vi "TEST.vi"() -> ()   [LabVIEW 2015, in "Copy of Untitled Library 1.lvlib"]
uses:
  Copy of Untitled Library 1.lvlib
  <userlib>/origin_lib_main/userlogin_lib/Control/Queue and Caller MSG.ctl
  Controls/Control 1.ctl
  <vilib>/addons/database/Connection.llb/DB Tools Open Connec (String).vi
  API/Init Module.vi
  API/Get Open batch .vi
  Main.vi
  <vilib>/addons/database/NI_Database_API.lvlib
panel:
  out "subarray":string[](array[string])
  in  "Get Open Batch data":bool
  out "Batch Data 3":T1
  out "Module Number 2":dbl
  out "Product name":string
  out "UI Controllers":string[](array[string])
  out "Enum":T2(ring)
  in  "stop 2":bool
  in  "Init":bool
  in  "Module Number":dbl=1.0
  in  "Main":bool
  in  "stop":bool
  out "error out":errorcluster
  in  "UI COnfiguration  2":T4
  # "QUEUE"
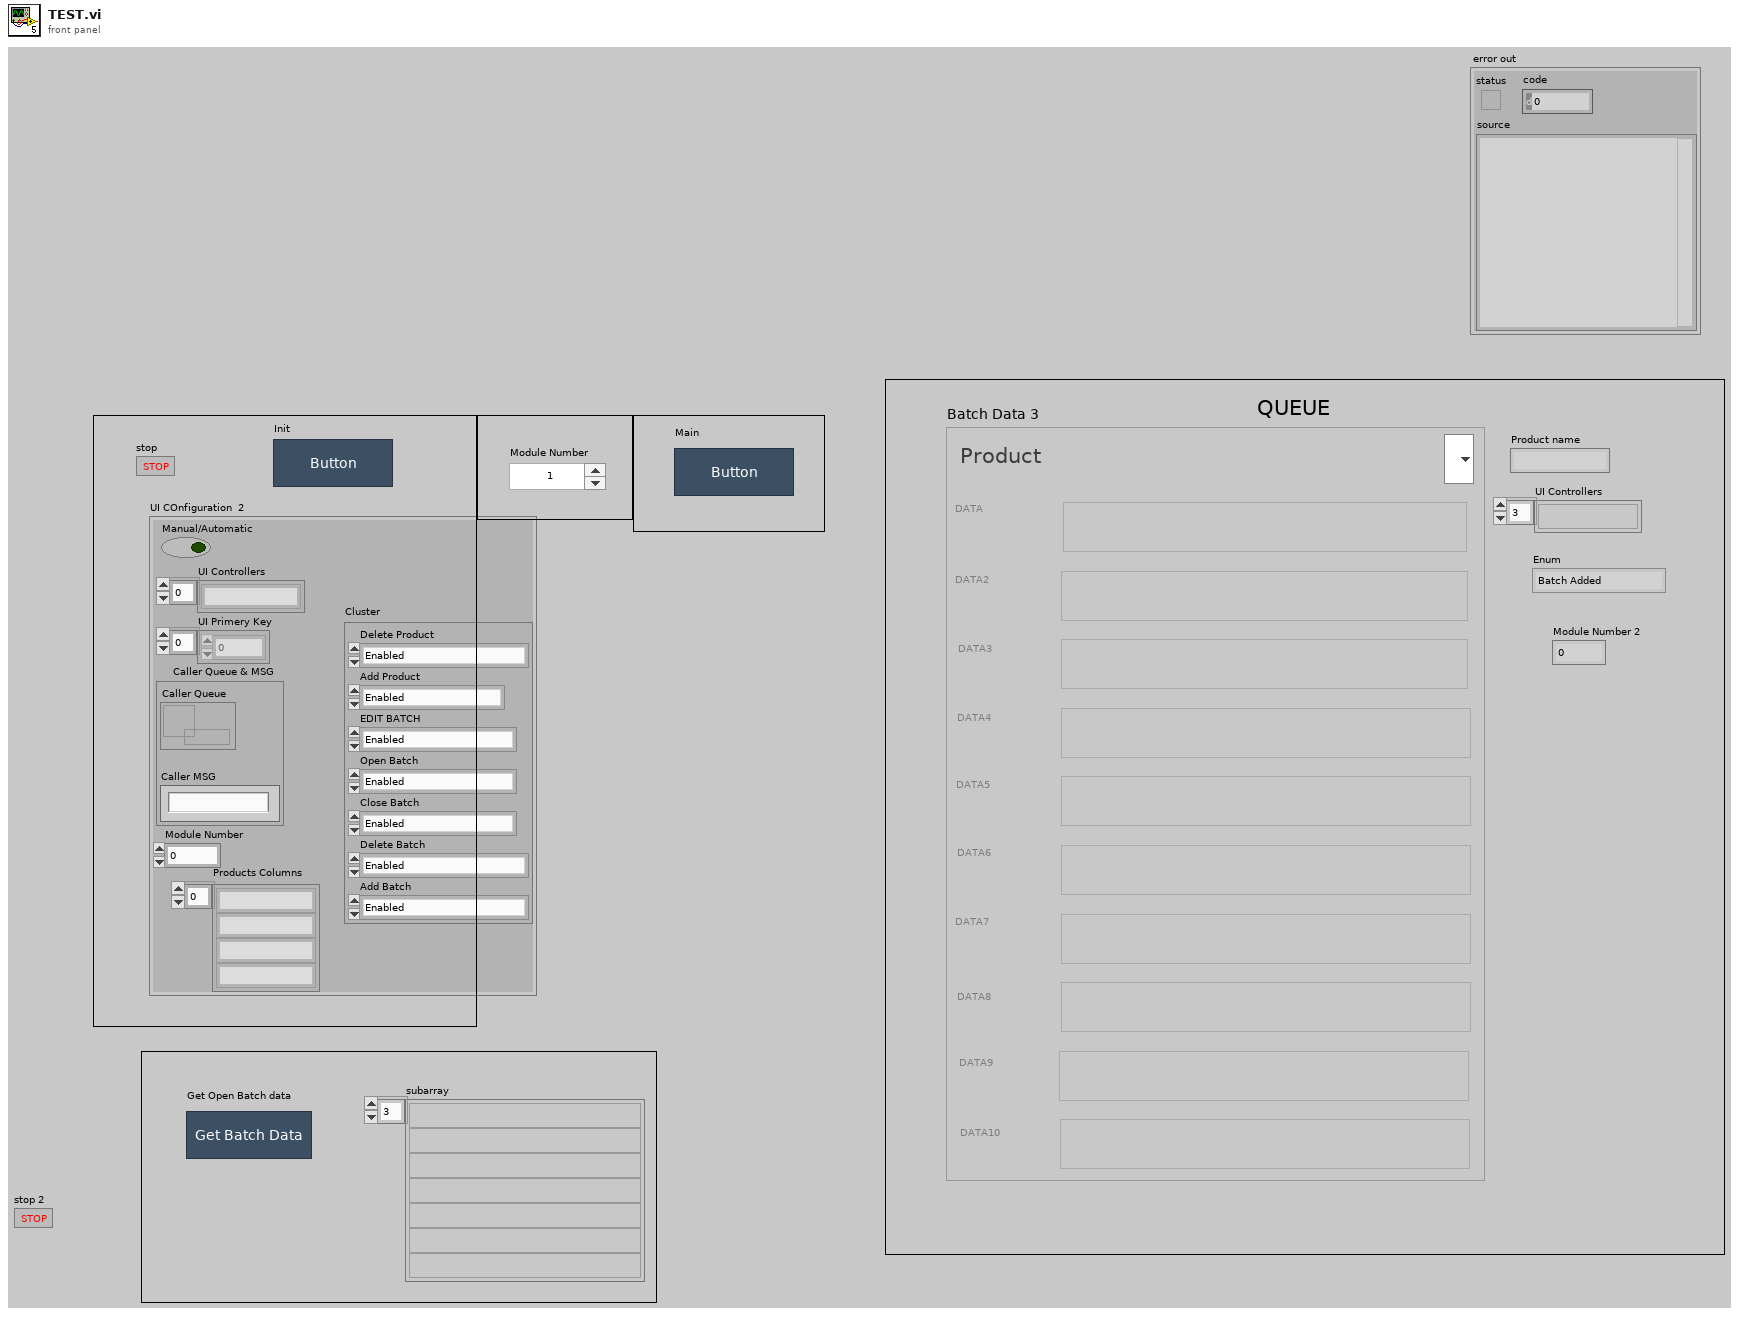
[diagram p1: front panel]
types:
  T1 = typedef "Copy of Untitled Library 1.lvlib/Control 1.ctl" = cluster{"DATA":string, "DATA 2":string, "DATA 3":string, "DATA 4":string, "DATA 5":string, "DATA 6":string, "DATA 7":string, "DATA 8":string, "DATA 9":string, "DATA 10":string, "Product":string}
  T2 = enum16{"Batch Added", "Batch Deleted", "Batch Opened", "Batch Closed", "Batch Edited", "new Product Added", "Product deleted "}
  T3 = typedef "Queue and Caller MSG.ctl" = cluster{"Caller Queue":refnum<queue>, "Caller MSG":string}
  T4 = cluster{"Manual/Automatic":bool, "UI Controllers ":string[], "UI Primery Key ":dbl[], "Caller Queue & MSG":T3, "Module Number":dbl, "Products Columns":string[], "Cluster":cluster{"Delete Product":enum8{"Enabled", "Disabled", "Disabled and Grayed Out"}, "Add Product ":enum8{"Enabled", "Disabled", "Disabled and Grayed Out"}, "EDIT BATCH":enum8{"Enabled", "Disabled", "Disabled and Grayed Out"}, "Open Batch ":enum8{"Enabled", "Disabled", "Disabled and Grayed Out"}, "Close Batch":enum8{"Enabled", "Disabled", "Disabled and Grayed Out"}, "Delete Batch":enum8{"Enabled", "Disabled", "Disabled and Grayed Out"}, "Add Batch ":enum8{"Enabled", "Disabled", "Disabled and Grayed Out"}}}
  T5 = typedef "NI_Database_API.lvlib/Conn ObjectReference.ctl" = refnum<k1>
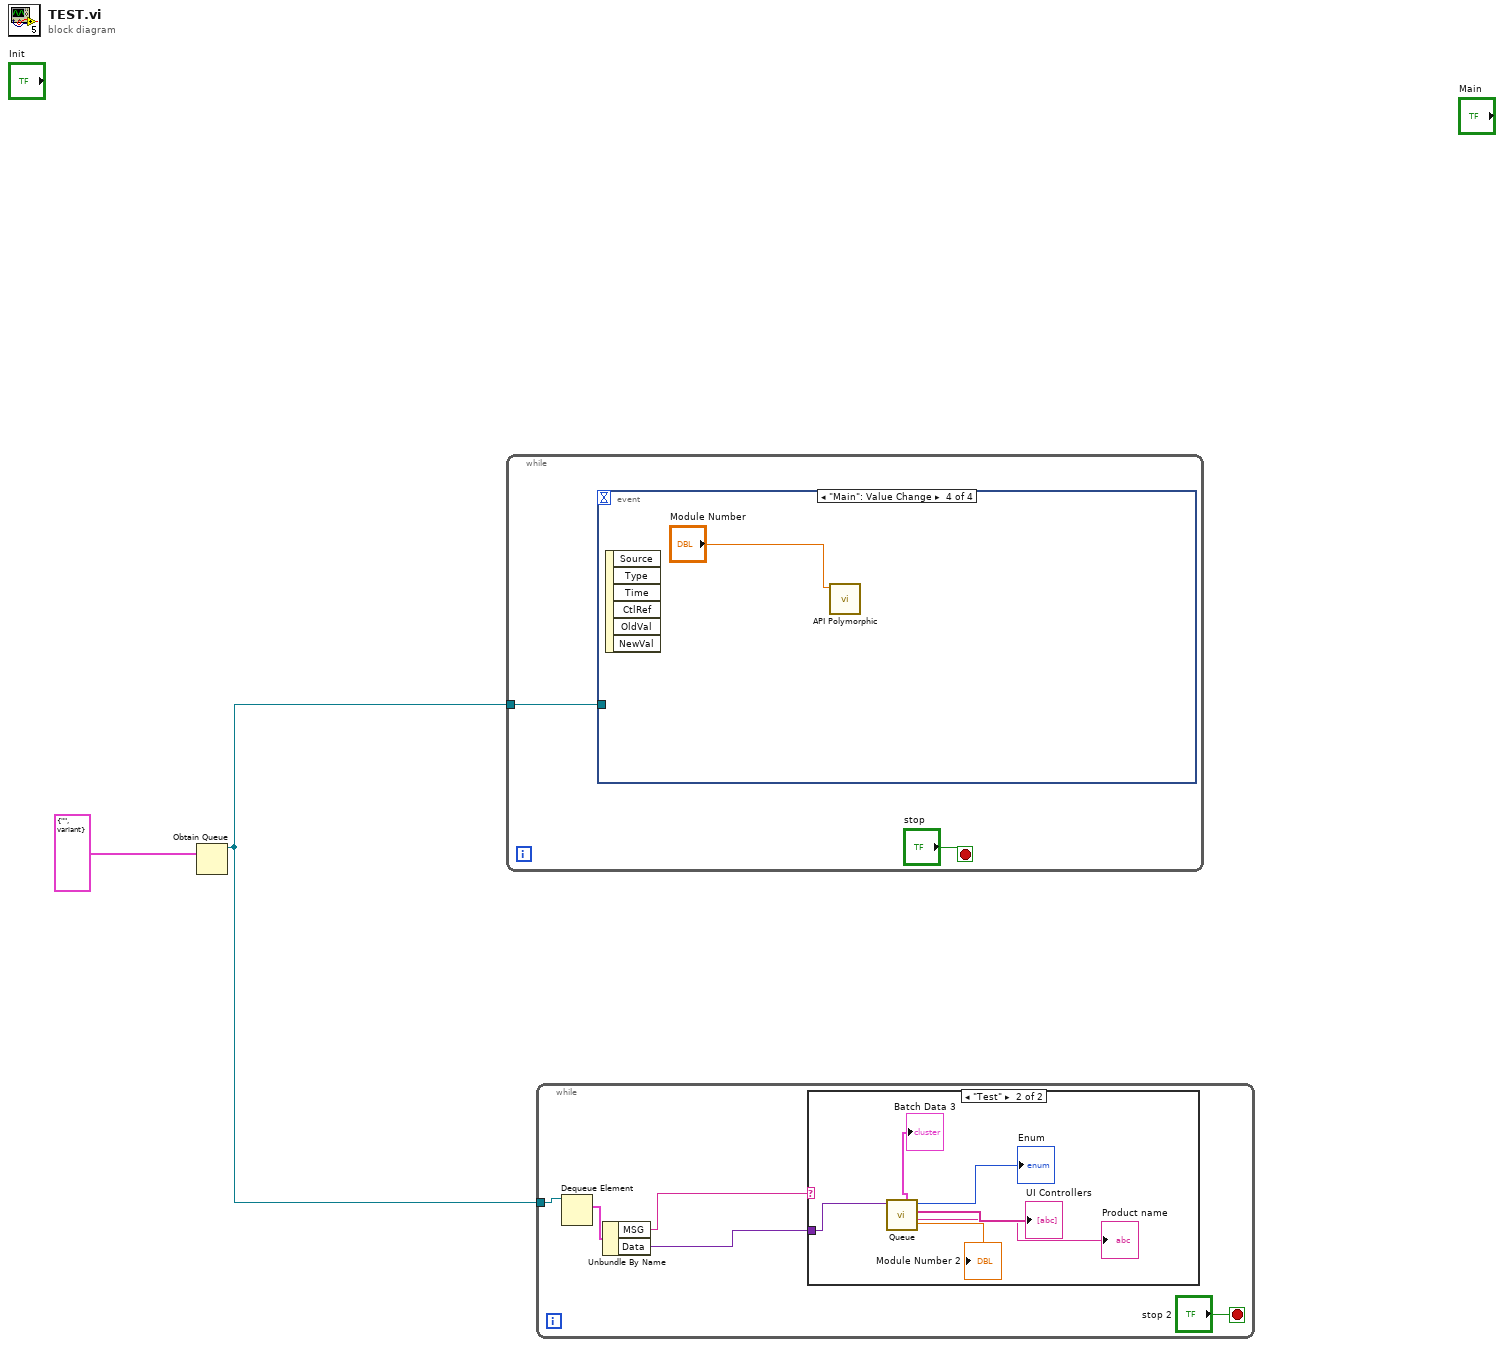
[diagram p0: block diagram]
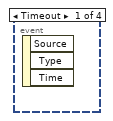
[diagram p3: hidden frame]
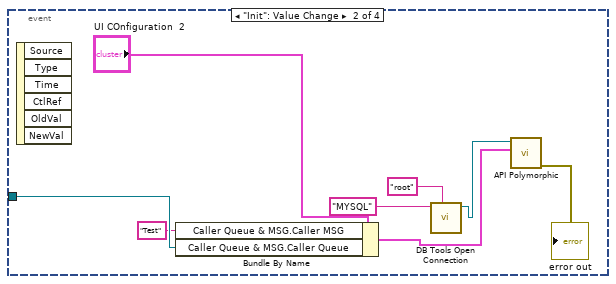
[diagram p4: hidden frame]
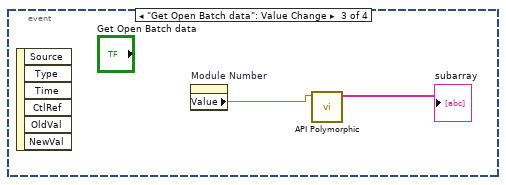
[diagram p5: hidden frame]
diagram:
  n1 = Obtain Queue(element data type=cluster{"MSG":string, "Data":variant} {"MSG"="", "Data"=variant}) -> (queue out=w1:refnum<queue>)  [unwired: 4 in, 2 out]
  n2 = while {
    tunnel: w1 -> [w3]
    stop <- "stop" stop-if-true
    n3 = event shown="[3] \"Main\": Value Change" {
      selector: _ -> [_ _ _ _]
      dyn-events: _ -> [_ _ _ _]
      timeout: _ -> [_ _ _ _]
      tunnel: w3 -> [_ w9 _ _]
      event Timeout {
        n4 = event-data() -> ()  [unwired: 1 in, 3 out]
      }
      event "Init": Value Change {
        n5 = event-data() -> ()  [unwired: 1 in, 6 out]
        n6 = Bundle By Name(cluster="UI COnfiguration  2", "Caller Queue & MSG.Caller MSG"="Test", "Caller Queue & MSG.Caller Queue"=w9) -> (w6:T4)
        n7 = call-poly <vilib>:"DB Tools Open Connection.vi"("userID"="root", "connection information"="MYSQL" ("userID")) -> ("connection reference"=w7:T5)  [unwired: 6 in, 1 out]
        n8 = call-poly "API Polymorphic.vi"("UI COnfiguration  3"=w6, "DB Reference In"=w7) -> ("error out"=→"error out":errorcluster)  [unwired: 9 in]
      }
      event "Get Open Batch data": Value Change {
        n9 = event-data() -> ()  [unwired: 1 in, 6 out]
        n10 = property on="Module Number" class="DigNum (strict)"() -> ("Value"=w14:dbl)  [unwired: 2 in, 2 out]
        n11 = call-poly "API Polymorphic.vi"("Module Number  2"=w14) -> ("subarray"=→"subarray":string[])  [unwired: 9 in, 1 out]
      }
      event "Main": Value Change {
        n12 = event-data() -> ()  [unwired: 1 in, 6 out]
        n13 = call-poly "API Polymorphic.vi"("Module Number"="Module Number") -> ()  [unwired: 11 in]
      }
    }
  }
  n14 = while {
    tunnel: w1 -> [w20]
    stop <- "stop 2" stop-if-true
    n15 = Dequeue Element(queue=w20) -> (element=w19:cluster{"MSG":string, "Data":variant})  [unwired: 2 in, 3 out]
    n16 = Unbundle By Name(w19) -> ("MSG"=w18:string, "Data"=w17:variant)
    n17 = case shown="\"Test\"" w18 {
      tunnel: w17 -> [_ w26]
      frame "False", Default {
      }
      frame "Test" {
        n18 = call "Queue.vi"("Data"=w26) -> ("Product name"=→"Product name":string, "UI Controllers"=→"UI Controllers":string[], "Enum"=→"Enum":T2, "Module Number"=→"Module Number 2":dbl, "Batch Data 3"=→"Batch Data 3":T1)  [unwired: 5 in, 1 out]
      }
    }
  }
